vi "finename.vi"() -> ()   [LabVIEW 2015]
panel:
  out "Signals 2":dbl
  out "Signals":dbl
  out "afterpath":path
  out "beforepath":path
  in  "isbefore":bool
  in  "stop":bool
  in  "Numeric":dbl
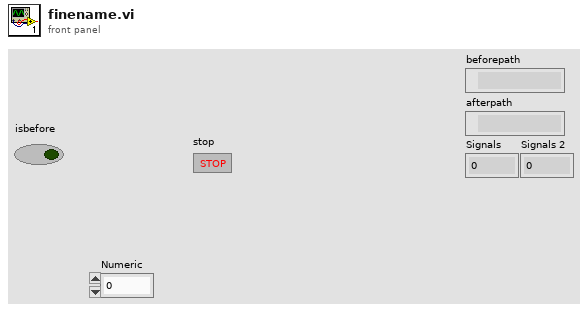
[diagram p1: front panel]
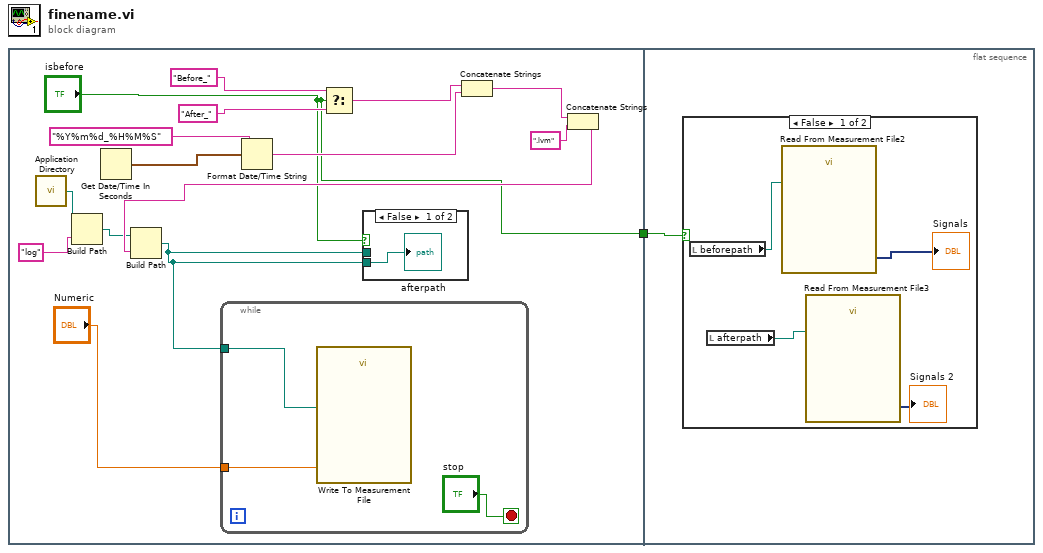
[diagram p0: block diagram]
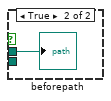
[diagram p2: hidden frame]
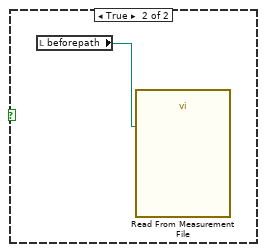
[diagram p3: hidden frame]
diagram:
  n1 = flat-sequence {
    tunnel: ["isbefore"] -> w1
    tunnel: w1 -> [w22]
    frame #0 {
      n2 = call <vilib>:"Application Directory.vi"() -> ("Application Directory"=w5:path)
      n3 = Build Path(base path=w5, name or relative path="log") -> (appended path=w4:path)
      n4 = Get Date/Time In Seconds() -> (seconds since 1Jan1904=w13:timestamp)
      n5 = Format Date/Time String(time format string (%c)="%Y%m%d_%H%M%S", seconds (now)=w13) -> (date/time string=w15:string)  [unwired: 1 in]
      n6 = Select(t="Before_", s="isbefore", f="After_") -> (s? t:f=w14:string)
      n7 = Concatenate Strings(w14, w15) -> (w16:string)
      n8 = Concatenate Strings(w16, ".lvm") -> (w8:string)
      n9 = Build Path(base path=w4, name or relative path=w8) -> (appended path=w2:path)
      n10 = while {
        tunnel: w2 -> [w20]
        tunnel: "Numeric" -> [w19]
        stop <- "stop" stop-if-true
        n11 = call "Write To Measurement File"("Signals"=w19, "Filename"=w20) -> ()  [unwired: 15 in, 3 out]
      }
      n12 = case shown="False" "isbefore" {
        tunnel: w2 -> [_ w18]
        tunnel: w2 -> [w17 _]
        frame False {
          "afterpath" <- w17
        }
        frame True {
          "beforepath" <- w18
        }
      }
    }
    frame #1 {
      n13 = case shown="False" w22 {
        frame False {
          n14 = local read "beforepath"() -> (w25:path)
          n15 = local read "afterpath"() -> (w26:path)
          n16 = call "Read From Measurement File2"("Filename"=w25) -> ("Signals"=→"Signals":dynamicdata)  [unwired: 5 in, 5 out]
          n17 = call "Read From Measurement File3"("Filename"=w26) -> ("Signals"=→"Signals 2":dynamicdata)  [unwired: 5 in, 5 out]
        }
        frame True {
          n18 = local read "beforepath"() -> (w27:path)
          n19 = call "Read From Measurement File"("Filename"=w27) -> ()  [unwired: 5 in, 6 out]
        }
      }
    }
  }
